vi "configureAcquisition_action.vi"(0 "HGF_ImaqFg":refnum<class "HGF_ImaqFg.lvclass">, 2 "Continuous?":enum16{"One-Shot", "Continuous"}(ring)=enum."Continuous", 3 "Number of buffers":u32, 5 "error in (no error)":errorcluster, 6 "Region of Interest":i32[](array[numeric]), 7 "Memory Location":enum16{"System", "Onboard"}(ring), 8 "Buffer Parameters":cluster{"Skip Count":u32, "Channel":i32}[](array[cluster]), 9 "Image Array":T1[](array[typedef])) -> (14 "dup HGF_ImaqFg":refnum<class "HGF_ImaqFg.lvclass">, 19 "error out":errorcluster)   [LabVIEW 2014, in "HGF_IMAQ.lvlib" / "HGF_ImaqFg.lvclass"]
doc: "Configures a low-level acquisition previously opened with IMAQdx Open Camera VI. Specify the acquisition type with the Continuous? and Number of Buffers parameters. \n\nSnap: Continuous = 0; Buffer Count = 1 \nSequence: Continuous = 0; Buffer Count > 1 \nGrab: Continuous = 1; Buffer Count > 1"
uses:
  HGF_ImaqFg.lvclass
  <vilib>/vision/Image Controls.llb/IMAQ Image.ctl
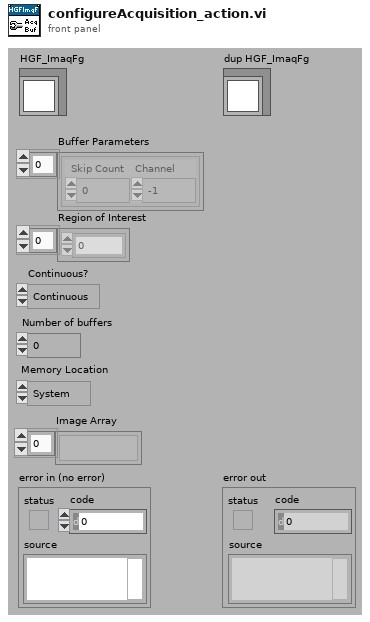
[diagram p1: front panel]
types:
  T1 = typedef "IMAQ Image.ctl" = refnum<image>
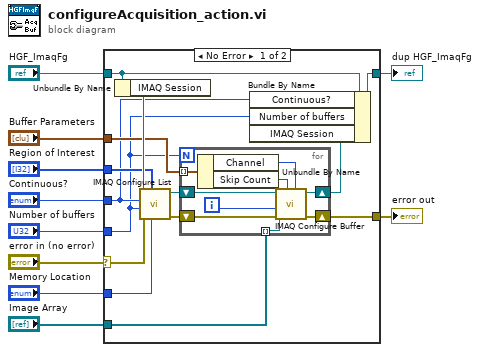
[diagram p0: block diagram]
diagram:
  n1 = case shown="No Error" "error in (no error)" {
    selector: "error in (no error)" -> [w13 w34]
    tunnel: "Continuous?" -> [w12 _]
    tunnel: "Memory Location" -> [w23 _]
    tunnel: "Region of Interest" -> [w22 _]
    tunnel: "Image Array" -> [w19 _]
    tunnel: "Number of buffers" -> [w11 _]
    tunnel: "Buffer Parameters" -> [w18 _]
    tunnel: "HGF_ImaqFg" -> [w17 w35]
    tunnel: [w15 w35] -> w3
    tunnel: [w14 w34] -> w2
    frame No Error {
      n2 = Unbundle By Name(w17) -> ("IMAQ Session"=w24:refnum<k11>)
      n3 = call <vilib>:"IMAQ Configure List.vi"("Memory Location"=w23, "Region of interest"=w22, "error in (no error)"=w13, "Number of buffers"=w11, "Continuous?"=w12, "IMAQ Session In"=w24) -> ("error out"=w20:errorcluster, "IMAQ Session Out"=w21:refnum<k11>)  [unwired: 4 out]
      n4 = for {
        N: w11 -> [_]
        tunnel: w19 -> [w31] mode=indexing
        tunnel: w18 -> [w29] mode=indexing
        shift-right: [w26] -> w14
        shift-left: w20 -> [w32]
        shift-right: [w25] -> w16
        shift-left: w21 -> [w33]
        i -> [w30]
        n5 = Unbundle By Name(w29) -> ("Channel"=w27:i32, "Skip Count"=w28:u32)
        n6 = call <vilib>:"IMAQ Configure Buffer.vi"("Channel"=w27, "Skip Count"=w28, "error in (no error)"=w32, "Buffer Number"=w30, "Image In"=w31, "IMAQ Session In"=w33) -> ("error out"=w26:errorcluster, "IMAQ Session Out"=w25:refnum<k11>)  [unwired: 4 out]
      }
      n7 = Bundle By Name(cluster=w17, "Continuous?"=w12, "Number of buffers"=w11, "IMAQ Session"=w16) -> (w15:refnum<class "HGF_ImaqFg.lvclass">)
    }
    frame Error {
    }
  }
  "error out" <- w2
  "dup HGF_ImaqFg" <- w3
